vi "禹山获取系列号.vi"(7 "探头":T1(ring), 8 "error in (no error)":errorcluster caption="错误输入（无错误）", 11 "MB session in":refnum<class "MB_Master.lvclass">) -> (0 "error out":errorcluster caption="错误输出", 2 "SN":string, 3 "MB session out":refnum<class "MB_Master.lvclass">)   [LabVIEW 2016, in "斯坦道多参数.lvlib"]
uses:
  <vilib>/Plasmionique/MB Master/MB_Master/MB_Master.lvclass
  <vilib>/Plasmionique/MB Master/MB Master.lvlib
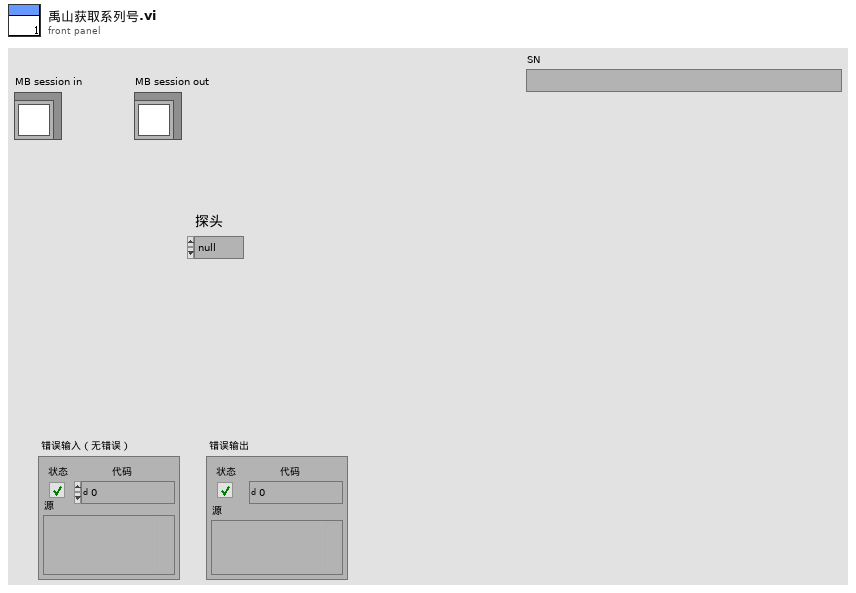
[diagram p1: front panel]
types:
  T1 = enum16{"null", "pH", "DO", "浊度", "电导率", "叶绿素a", "DO2"}
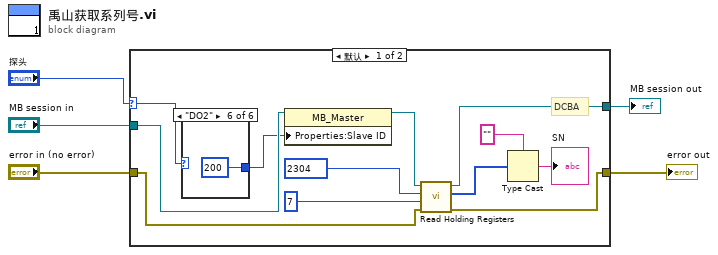
[diagram p0: block diagram]
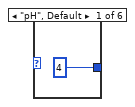
[diagram p2: hidden frame]
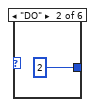
[diagram p3: hidden frame]
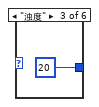
[diagram p4: hidden frame]
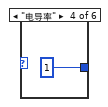
[diagram p5: hidden frame]
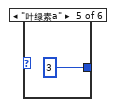
[diagram p6: hidden frame]
diagram:
  n1 = case shown="默认" "探头" {
    selector: "探头" -> [w6 _]
    tunnel: "error in (no error)" -> [w15 w24]
    tunnel: "MB session in" -> [w13 w25]
    tunnel: [w8 w25] -> w3
    tunnel: [w7 w24] -> w2
    frame Default {
      # "DCBA"
      n2 = case shown="\"DO2\"" w6 {
        tunnel: [u16 4 ("y") u16 2 ("y") u16 20 ("y") u16 1 ("y") u16 3 ("y") u16 200 ("y")] -> w9
        frame "pH", Default {
        }
        frame "DO" {
        }
        frame "浊度" {
        }
        frame "电导率" {
        }
        frame "叶绿素a" {
        }
        frame "DO2" {
        }
      }
      n3 = property class="MB_Master"(reference=w13, "Properties:Slave ID"=w9) -> (reference out=w14:refnum<class "MB_Master.lvclass">)  [unwired: 1 in, 1 out]
      n4 = call <vilib>:"Read Holding Registers.vi"("error in (no error)"=w15, "quantity"=u16 7, "starting address"=u16 2304, "MB session in"=w14) -> ("error out"=w7:errorcluster, "Registers"=w12:u16[], "MB session out"=w8:refnum<class "MB_Master.lvclass">)  [unwired: 5 in]
      n5 = Type Cast(type="", x=w12) -> (*(type *) &x=→"SN":string)
    }
    frame "null" {
    }
  }
  "MB session out" <- w3
  "error out" <- w2
